vi "APC_9056_ForceArraySize16.vi"(1 "ArrayIn":dbl[](array[numeric]) format="%0.2f") -> (0 "ArraOut":dbl[](array[numeric]))   [LabVIEW 2020]
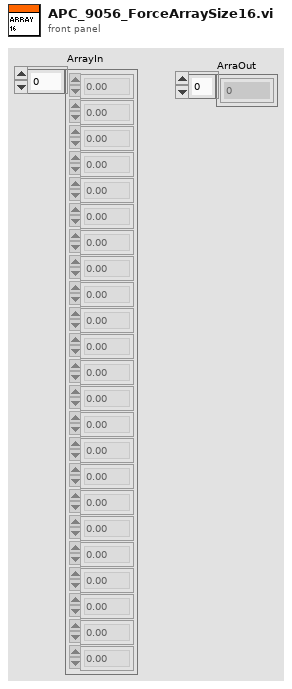
[diagram p1: front panel]
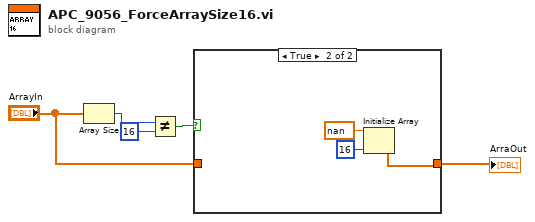
[diagram p0: block diagram]
diagram:
  n1 = Array Size(array="ArrayIn") -> (size(s)=w4:i32)
  n2 = Not Equal?(x=w4, y=16) -> (x != y?=w5:bool)
  n3 = case shown="True" w5 {
    tunnel: [w6 w9] -> w1
    tunnel: "ArrayIn" -> [w6 _]
    frame False {
    }
    frame True {
      n4 = Initialize Array(nan ("element"), 16 ("dimension size")) -> (w9:dbl[])
    }
  }
  "ArraOut" <- w1
